vi "Read Pin Map Original.vi"(8 "error in (no error)":errorcluster, 11 "NI-DAQ in":refnum<class "NI-DAQ.lvclass">) -> (0 "error out":errorcluster, 2 "Pin Map":T1={"Region Valves"=[49, 52, 0, 0], "Extra Valves"=[[[0.0, 48.0, 0.0, 0.0, 0.0]]], "Tool Primary Valve"=51, "Tool Secondary Valve"=50, "Region Sensors"=[37, 41, 37], "Extra Sensors"=[[[36.0, 37.0, 0.0, 0.0]]], "Tool Primary Sensor"=39.0, "Tool Secondary Sensor"=38.0, "Compression Sensor"=31.0, "5V"=50, "Dispenser Sensor"=0.0}, 3 "NI-DAQ out":refnum<class "NI-DAQ.lvclass">)   [LabVIEW 2021, in "NI-DAQ.lvclass"]
uses:
  NI-DAQ.lvclass
  <vilib>/Utility/file.llb/Read Delimited Spreadsheet (DBL).vi
  I-O.lvclass
  Pin Map.ctl
panel:
  out "extra valves":i32[][][](array[numeric])
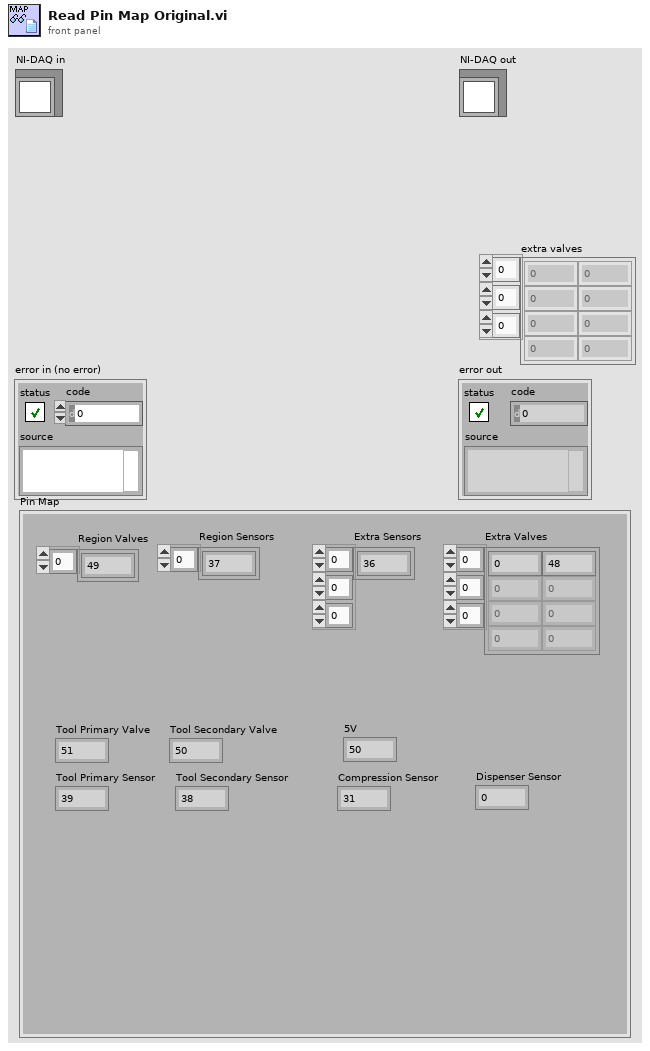
[diagram p1: front panel]
types:
  T1 = typedef "I-O.lvclass/Pin Map.ctl" = cluster{"Region Valves":i32[], "Extra Valves":dbl[][][], "Tool Primary Valve":i32, "Tool Secondary Valve":i32, "Region Sensors":i32[], "Extra Sensors":dbl[][][], "Tool Primary Sensor":dbl, "Tool Secondary Sensor":dbl, "Compression Sensor":dbl, "5V":i32, "Dispenser Sensor":dbl}
  T2 = typedef "File Paths.ctl" = cluster{"Glue Pattern Folder":path, "Carrier Tray Folder":path, "Pick Up Tool Fixture Folder":path, "Components Folder":path, "Bellows Tool Offset.txt":path, "Pick Up Tool Offset.txt":path, "Dispense Tip Offset.txt":path, "Log Files":path, "Gantry Assembly Map.txt":path, "Syringe and offset map.txt":path, "Controllers Folder":path, "Local dbase config":path}
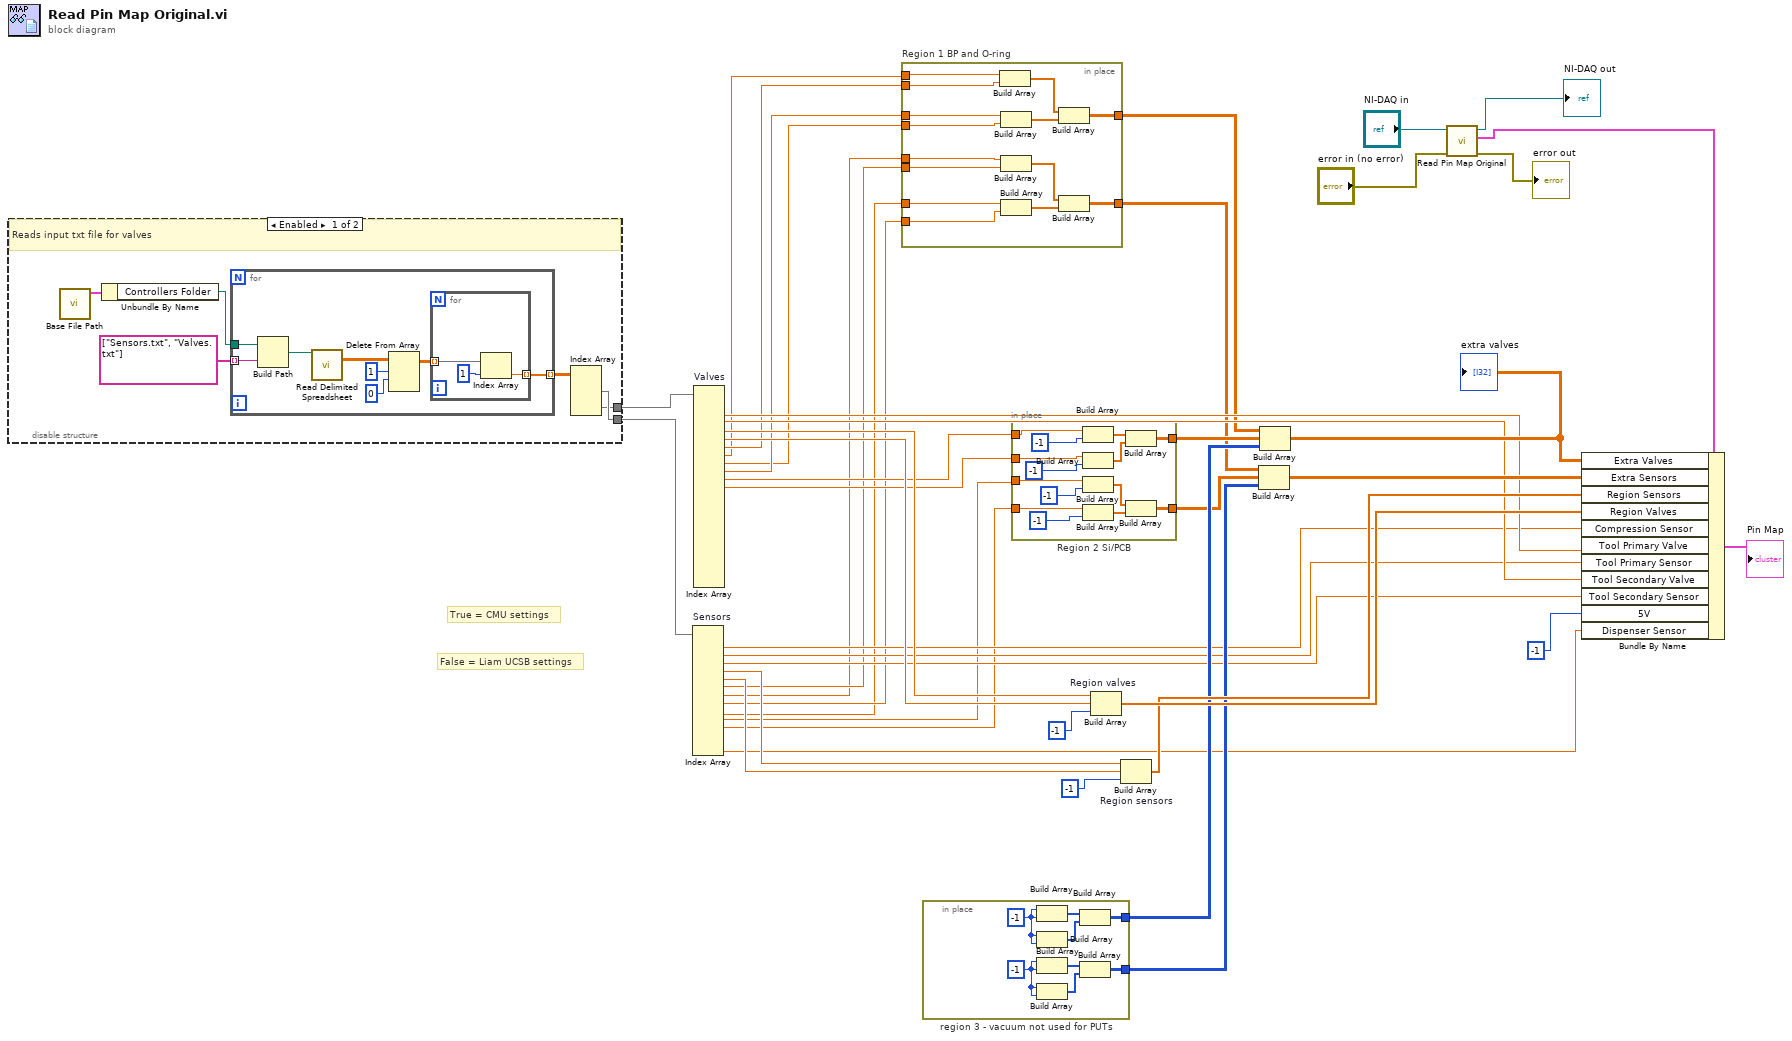
[diagram p0: block diagram]
diagram:
  # "False = Liam UCSB settings"
  # "True = CMU settings"
  n1 = disable-structure shown="Enabled" {
    disable-tunnel: [w45 _] -> w43
    disable-tunnel: [w44 _] -> w42
    frame Enabled {
      # "Reads input txt file for valves"
      n2 = call "Base File Path.vi"() -> ("Paths Out"=w49:T2)  [unwired: 11 in]
      n3 = Unbundle By Name(w49) -> ("Controllers Folder"=w47:path)
      n4 = for {
        tunnel: string[] ["Sensors.txt", "Valves.txt"] -> [w55] mode=indexing
        tunnel: w47 -> [w56]
        tunnel: [w50] -> w46 mode=indexing
        n5 = Build Path(base path=w56, name or relative path=w55) -> (appended path=w57:path)
        n6 = call-poly <vilib>:"Read Delimited Spreadsheet.vi"("file path (dialog if empty)"=w57) -> ("all rows"=w54:dbl[][])  [unwired: 9 in, 5 out]
        n7 = Delete From Array(array=w54, length=1, index (row)=0) -> (array with subset deleted=w51:dbl[][])  [unwired: 1 in, 1 out]
        n8 = for {
          tunnel: w51 -> [w60] mode=indexing
          tunnel: [w59] -> w50 mode=indexing
          n9 = Index Array(array=w60, index=1) -> (element=w59:dbl)
        }
      }
      n10 = Index Array(array=w46) -> (element #1=w45:dbl[], element #2=w44:dbl[])  [unwired: 4 in]
    }
    frame Disabled {
    }
  }
  n11 = Index Array "Sensors"(array=w43) -> (element #1=w16:dbl, element #2=w15:dbl, element #3=w14:dbl, element #4=w13:dbl, element #5=w12:dbl, element #6=w11:dbl, element #7=w10:dbl, element #8=w9:dbl, element #9=w8:dbl, element #10=w7:dbl, element #11=w6:dbl, element #14=w5:dbl)  [unwired: 14 in, 2 out]
  n12 = Index Array "Valves"(array=w42) -> (element #2=w26:dbl, element #3=w25:dbl, element #4=w24:dbl, element #5=w23:dbl, element #6=w22:dbl, element #7=w21:dbl, element #8=w19:dbl, element #9=w20:dbl, element #10=w18:dbl, element #11=w17:dbl)  [unwired: 23 in, 13 out]
  n13 = in-place "Region 1 BP and O-ring" {
    in-place-border: [w72] -> w4
    in-place-border: [w69] -> w2
    in-place-border: w22 -> [w68]
    in-place-border: w21 -> [w67]
    in-place-border: w20 -> [w66]
    in-place-border: w19 -> [w65]
    in-place-border: w11 -> [w64]
    in-place-border: w10 -> [w63]
    in-place-border: w9 -> [w62]
    in-place-border: w8 -> [w61]
    n14 = Build Array(w67, w68) -> (w74:dbl[])
    n15 = Build Array(w66, w65) -> (w73:dbl[])
    n16 = Build Array(w63, w64) -> (w71:dbl[])
    n17 = Build Array "Build Array"(w61, w62) -> (w70:dbl[])
    n18 = Build Array(w74, w73) -> (w72:dbl[][])
    n19 = Build Array "Build Array"(w71, w70) -> (w69:dbl[][])
  }
  n20 = in-place "region 3 - vacuum not used for PUTs" {
    in-place-border: [w79] -> w31
    in-place-border: [w76] -> w30
    w75 = -1
    w81 = -1
    n21 = Build Array(w81, w81) -> (w82:i32[])
    n22 = Build Array(w81, w81) -> (w80:i32[])
    n23 = Build Array(w75, w75) -> (w78:i32[])
    n24 = Build Array(w75, w75) -> (w77:i32[])
    n25 = Build Array(w82, w80) -> (w79:i32[][])
    n26 = Build Array(w78, w77) -> (w76:i32[][])
  }
  n27 = in-place "Region 2 Si/PCB" {
    in-place-border: [w94] -> w3
    in-place-border: [w91] -> w1
    in-place-border: w18 -> [w86]
    in-place-border: w17 -> [w85]
    in-place-border: w7 -> [w84]
    in-place-border: w6 -> [w83]
    n28 = Build Array(w86, -1) -> (w95:dbl[])
    n29 = Build Array(w85, -1) -> (w96:dbl[])
    n30 = Build Array(w84, -1) -> (w92:dbl[])
    n31 = Build Array(w83, -1) -> (w93:dbl[])
    n32 = Build Array(w95, w96) -> (w94:dbl[][])
    n33 = Build Array(w92, w93) -> (w91:dbl[][])
  }
  n34 = Build Array "Region valves"(w24, w23, -1) -> (w35:dbl[])
  n35 = Build Array "Region sensors"(w13, w12, -1) -> (w32:dbl[])
  n36 = Build Array(w2, w1, w30) -> (w28:dbl[][][])
  n37 = Build Array(w4, w3, w31) -> (w29:dbl[][][])
  "extra valves" <- w29
  n38 = call-parent "Read Pin Map Original.vi"("error in (no error)"="error in (no error)", "I-O in"="NI-DAQ in") -> ("error out"=→"error out":errorcluster, "Pin Map 2"=w37:T1, "I-O out"=→"NI-DAQ out":refnum<class "NI-DAQ.lvclass">)  [unwired: 7 in]
  n39 = Bundle By Name(cluster=w37, "Extra Valves"=w29, "Extra Sensors"=w28, "Region Sensors"=w32, "Region Valves"=w35, "Compression Sensor"=w16, "Tool Primary Valve"=w26, "Tool Primary Sensor"=w15, "Tool Secondary Valve"=w25, "Tool Secondary Sensor"=w14, "5V"=-1, "Dispenser Sensor"=w5) -> (→"Pin Map":T1)
